vi "DT3120_FG_SINGLE_FRAME_OPS.vi"(11 "OLT_FG_SINGLE_FRAME_OPS":u8[](array[numeric])) -> (1 "ops":T1, 3 "DoesSyncPassthru":bool)   [LabVIEW 2010]
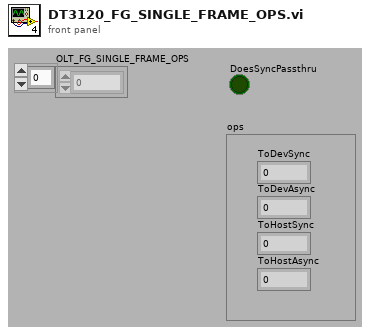
[diagram p1: front panel]
types:
  T1 = cluster{"ToDevSync":u32, "ToDevAsync":u32, "ToHostSync":u32, "ToHostAsync":u32}
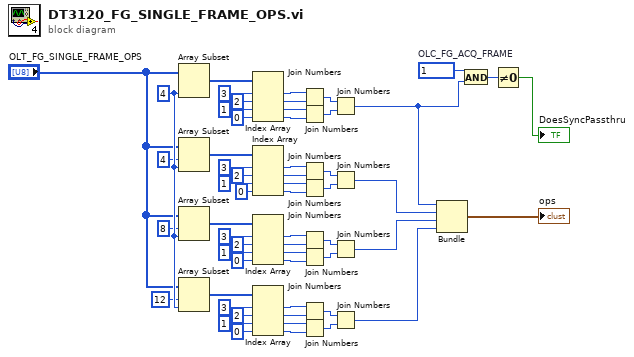
[diagram p0: block diagram]
diagram:
  w11 = 4 ("length")
  w57 = u32 1  # OLC_FG_ACQ_FRAME
  n1 = Array Subset(array="OLT_FG_SINGLE_FRAME_OPS", length=w11) -> (w52:u8[])  [unwired: 1 in]
  n2 = Array Subset(array="OLT_FG_SINGLE_FRAME_OPS", index=4, length=w11) -> (w41:u8[])
  n3 = Array Subset(array="OLT_FG_SINGLE_FRAME_OPS", index=8, length=w11) -> (w30:u8[])
  n4 = Array Subset(array="OLT_FG_SINGLE_FRAME_OPS", index=12, length=w11) -> (w19:u8[])
  n5 = Index Array(array=w52, index #1=3 ("index"), index #2=2 ("index"), index #3=1 ("index"), index #4=0 ("index")) -> (element #1=w51:u8, element #2=w50:u8, element #3=w49:u8, element #4=w48:u8)
  n6 = Index Array(array=w41, index #1=3 ("index"), index #2=2 ("index"), index #3=1 ("index"), index #4=0 ("index")) -> (element #1=w40:u8, element #2=w39:u8, element #3=w38:u8, element #4=w37:u8)
  n7 = Index Array(array=w30, index #1=3 ("index"), index #2=2 ("index"), index #3=1 ("index"), index #4=0 ("index")) -> (element #1=w29:u8, element #2=w28:u8, element #3=w27:u8, element #4=w26:u8)
  n8 = Index Array(array=w19, index #1=3 ("index"), index #2=2 ("index"), index #3=1 ("index"), index #4=0 ("index")) -> (element #1=w18:u8, element #2=w17:u8, element #3=w16:u8, element #4=w15:u8)
  n9 = Join Numbers(hi=w51, lo=w50) -> ((hi.lo)=w47:u16)
  n10 = Join Numbers(hi=w49, lo=w48) -> ((hi.lo)=w46:u16)
  n11 = Join Numbers(hi=w40, lo=w39) -> ((hi.lo)=w36:u16)
  n12 = Join Numbers(hi=w38, lo=w37) -> ((hi.lo)=w35:u16)
  n13 = Join Numbers(hi=w29, lo=w28) -> ((hi.lo)=w25:u16)
  n14 = Join Numbers(hi=w27, lo=w26) -> ((hi.lo)=w24:u16)
  n15 = Join Numbers(hi=w18, lo=w17) -> ((hi.lo)=w14:u16)
  n16 = Join Numbers(hi=w16, lo=w15) -> ((hi.lo)=w13:u16)
  n17 = Join Numbers(hi=w47, lo=w46) -> ((hi.lo)=w1:u32)
  n18 = Join Numbers(hi=w36, lo=w35) -> ((hi.lo)=w6:u32)
  n19 = Join Numbers(hi=w25, lo=w24) -> ((hi.lo)=w5:u32)
  n20 = Join Numbers(hi=w14, lo=w13) -> ((hi.lo)=w4:u32)
  n21 = Bundle(w1, w6, w5, w4) -> (→"ops":cluster{u32, u32, u32, u32})  [unwired: 1 out]
  n22 = And(x=w57, y=w1) -> (x .and. y?=w56:u32)
  n23 = Not Equal To 0?(x=w56) -> (x != 0?=→"DoesSyncPassthru":bool)
